vi "Example Low Level.vi"() -> ()   [LabVIEW 2019]
uses:
  lib/labview_json.lvlib
panel:
  out "JSON out 2":string
  out "error out":errorcluster
  out "JSON out":string
  out "Exists?":bool
  in  "Root Path ([]=Root)":string[](array[string])
  in  "JSON in 2":string
  in  "JSON in":string
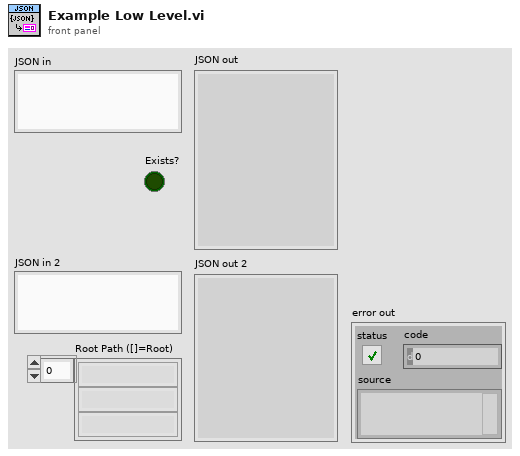
[diagram p1: front panel]
types:
  T1 = typedef "labview_json.lvlib/Element.ctl" = cluster{"Key":string, "Type":T2, "Value":variant}
  T2 = typedef "labview_json.lvlib/Element Type.ctl" = enum8{"NULL", "BOOL", "INT", "UINT", "FLOAT", "STRING", "ARRAY", "OBJECT", "SKIP"}
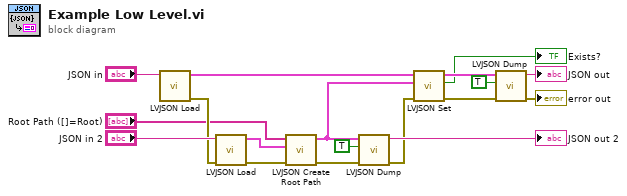
[diagram p0: block diagram]
diagram:
  n1 = call "LVJSON Load.vi"("JSON in"="JSON in") -> ("error out"=w14:errorcluster, "Root Element out"=w16:T1)  [unwired: 8 in, 1 out]
  n2 = call "LVJSON Load.vi"("error in (no error)"=w14, "JSON in"="JSON in 2") -> ("error out"=w7:errorcluster, "Root Element out"=w3:T1)  [unwired: 7 in, 1 out]
  n3 = call "LVJSON Create Root Path.vi"("error in (no error)"=w7, "Element in"=w3, "Root Path"="Root Path ([]=Root)") -> ("error out"=w6:errorcluster, "Root Element out"=w1:T1)  [unwired: 7 in]
  n4 = call "LVJSON Dump.vi"("error in (no error)"=w6, "Pretty Print? (F)"=TRUE, "Root Element in"=w1) -> ("error out"=w5:errorcluster, "JSON out"=→"JSON out 2":string)  [unwired: 6 in, 1 out]
  n5 = call "LVJSON Set.vi"("error in (no error)"=w5, "Root Element to Merge"=w1, "Root Element in"=w16) -> ("error out"=w4:errorcluster, "Exists?"=→"Exists?":bool, "Root Element out"=w15:T1)  [unwired: 6 in]
  n6 = call "LVJSON Dump.vi"("error in (no error)"=w4, "Pretty Print? (F)"=TRUE, "Root Element in"=w15) -> ("error out"=→"error out":errorcluster, "JSON out"=→"JSON out":string)  [unwired: 6 in, 1 out]
